vi "0_Dataset_Converter(CIFAR10).vi"() -> ()   [LabVIEW 2020]
uses:
  <vilib>/Utility/file.llb/Read Delimited Spreadsheet (string).vi
panel:
  out "error out":errorcluster
  out "Labels":string[](array[string])=["airplane", "automobile", "bird", "cat", "deer", "dog", "frog", "horse", "ship", "truck", ""]
  in  "Destination Path (Train and Test)":path=path "D:/DNN/CIFAR-10_Images"
  in  "CIFAR Path":path=path "D:/DNN/cifar-10-batches-bin"
  # "Overview:\nThis is a helper VI to convert CIFAR binary dataset into individual images, organized into separate folders based on their labels.\nInstructions:\n1. Download the CIFAR-10 binary version dataset from https://www.cs.toronto.edu/~kriz/cifar.html\n2. After downloading, extract the \"cifar-10-binary.tar.gz\" file, which will generate several files like \"data_batch_1.bin\", \n\"data_batch_2.bin\", ..., \"test_batch.bin\", and batches.meta.txt\".\n3. Set the \"CIFAR Path\"  to the folder where the files are extracted.\n3. Set the \"Destination Path (Train and Test)\" to where the images will be saved. \n4. Run the VI.\n5. Observe the content in the Destination folder."
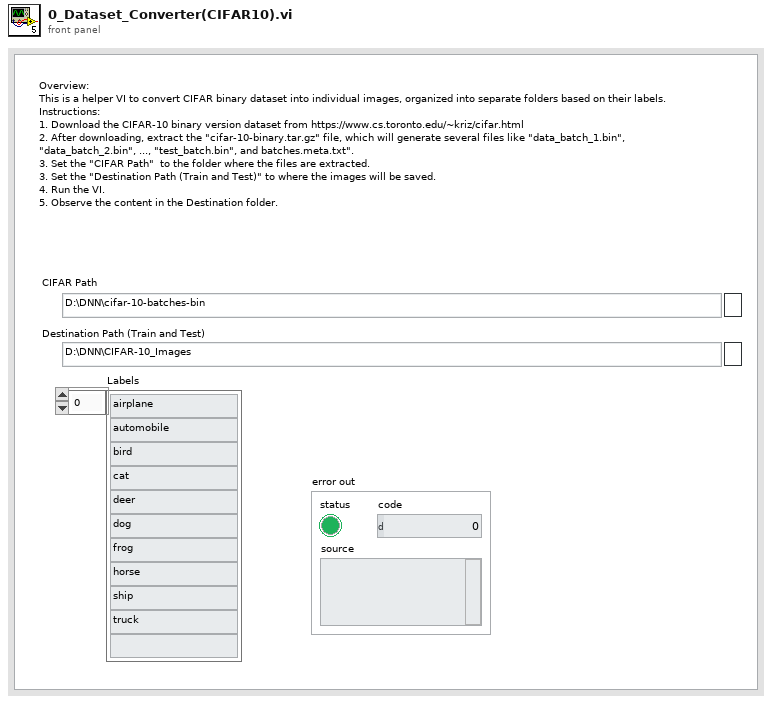
[diagram p1: front panel]
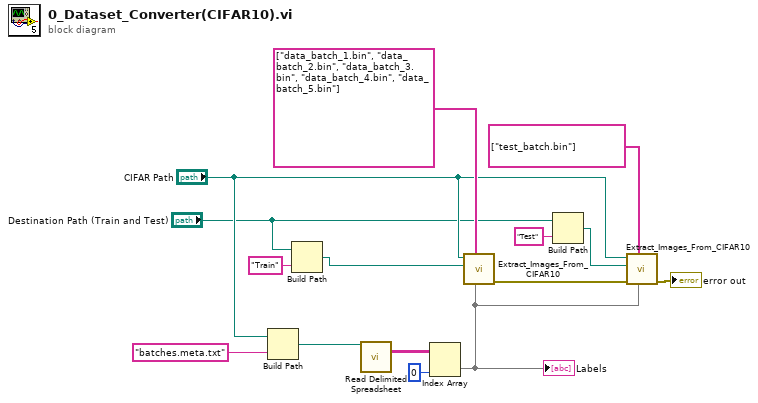
[diagram p0: block diagram]
diagram:
  n1 = Build Path(base path="CIFAR Path", name or relative path="batches.meta.txt") -> (appended path=w12:path)
  n2 = Build Path(base path="Destination Path (Train and Test)", name or relative path="Train") -> (appended path=w8:path)
  n3 = call-poly <vilib>:"Read Delimited Spreadsheet.vi"("file path (dialog if empty)"=w12) -> ("all rows"=w11:string[][])  [unwired: 9 in, 5 out]
  n4 = Index Array(array=w11, index (col)=0 ("disabled index (col)")) -> (element=w9:string[])  [unwired: 1 in]
  "Labels" <- w9
  n5 = call "Extract_Images_From_CIFAR10.vi"("Labels"=w9, "File Names"=string[] ["data_batch_1.bin", "data_batch_2.bin", "data_batch_3.bin", "data_batch_4.bin", "data_batch_5.bin"], "Destination Folder Path"=w8, "CIFAR Path"="CIFAR Path") -> ("error out"=w3:errorcluster)  [unwired: 7 in]
  n6 = Build Path(base path="Destination Path (Train and Test)", name or relative path="Test") -> (appended path=w4:path)
  n7 = call "Extract_Images_From_CIFAR10.vi"("Labels"=w9, "File Names"=string[] ["test_batch.bin"] ("pattern"), "error in"=w3, "Destination Folder Path"=w4, "CIFAR Path"="CIFAR Path") -> ("error out"=→"error out":errorcluster)  [unwired: 6 in]
